vi "Reset.vi"(8 "error in (no error)":errorcluster, 11 "NiPxi6123 in":refnum<class "NiPxi6123.lvclass">) -> (0 "error out":errorcluster, 3 "NiPxi6123 out":refnum<class "NiPxi6123.lvclass">)   [LabVIEW 2014, in "SamplerPlugins.lvlib" / "NiPxi6123.lvclass"]
uses:
  NiPxi6123.lvclass
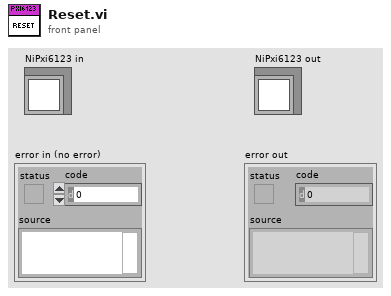
[diagram p1: front panel]
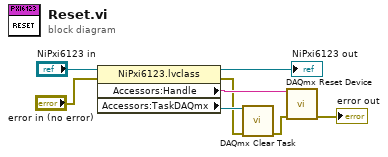
[diagram p0: block diagram]
diagram:
  n1 = property class="NiPxi6123.lvclass"(reference="NiPxi6123 in", error in="error in (no error)") -> (reference out=→"NiPxi6123 out":refnum<class "NiPxi6123.lvclass">, error out=w2:errorcluster, "Accessors:Handle"=w6:string, "Accessors:TaskDAQmx"=w3:refnum<k21>)
  n2 = call <vilib>:"DAQmx Clear Task.vi"("task in"=w3, "error in"=w2) -> ("error out"=w1:errorcluster)  [unwired: 13 in]
  n3 = call <vilib>:"DAQmx Reset Device.vi"("device in"=w6, "error in"=w1) -> ("error out"=→"error out":errorcluster)  [unwired: 13 in]
